vi "Delta Tiime.set.vi"(8 "error in (no error)":errorcluster, 10 "Delta Tiime":u32, 11 "midi-file-event in":refnum<class "midi-file-event.lvclass">) -> (0 "error out":errorcluster, 3 "midi-file-event out":refnum<class "midi-file-event.lvclass">)   [LabVIEW 2020, in "midi-file-event.lvclass"]
uses:
  midi-file-event.lvclass
  midi-file-event.lvclass/midi-file-event.ctl
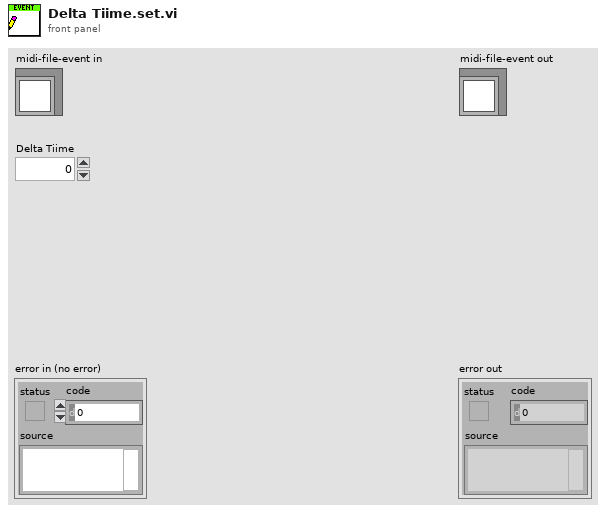
[diagram p1: front panel]
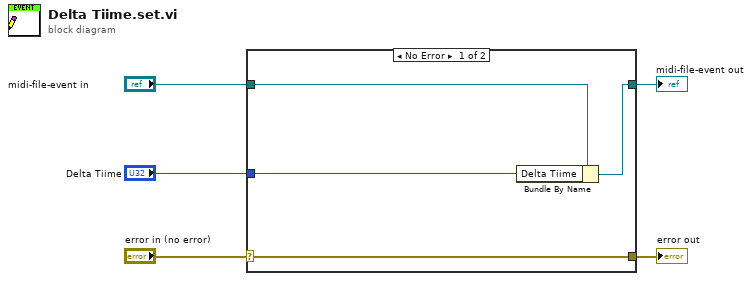
[diagram p0: block diagram]
diagram:
  n1 = case shown="No Error" "error in (no error)" {
    selector: "error in (no error)" -> [w9 w10]
    tunnel: [w9 w10] -> w4
    tunnel: [w7 w11] -> w2
    tunnel: "midi-file-event in" -> [w8 w11]
    tunnel: "Delta Tiime" -> [w6 _]
    frame No Error {
      n2 = Bundle By Name(cluster=w8, "Delta Tiime"=w6) -> (w7:refnum<class "midi-file-event.lvclass">)
    }
    frame Error {
    }
  }
  "error out" <- w4
  "midi-file-event out" <- w2
